vi "robot_ctrl.vi"(2 "Buttons":T1, 3 "Input":T3) -> (1 "Output":T2)   [LabVIEW 2024]
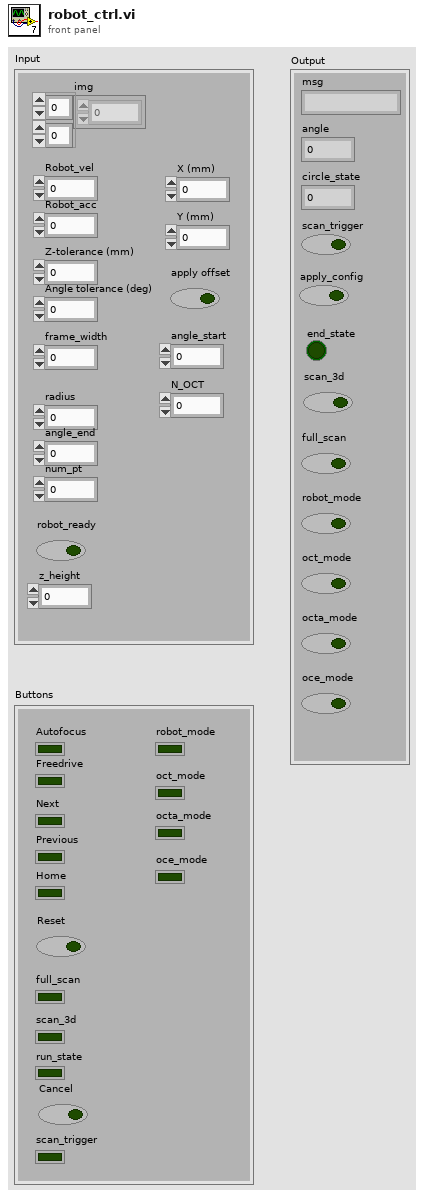
[diagram p1: front panel]
types:
  T1 = cluster{"Autofocus":bool, "Freedrive":bool, "Next":bool, "Previous":bool, "Home":bool, "Reset":bool, "full_scan":bool, "scan_3d":bool, "run_state":bool, "Cancel":bool, "scan_trigger":bool, "robot_mode":bool, "oct_mode":bool, "octa_mode":bool, "oce_mode":bool}
  T2 = cluster{"msg":string, "angle":dbl, "circle_state":i32, "scan_trigger":bool, "apply_config":bool, "end_state":bool, "scan_3d":bool, "full_scan":bool, "robot_mode":bool, "oct_mode":bool, "octa_mode":bool, "oce_mode":bool}
  T3 = cluster{"img":u8[][], "Robot_vel":dbl, "Robot_acc":dbl, "Z-tolerance (mm)":dbl, "Angle tolerance (deg)":dbl, "frame_width":i16, "radius":dbl, "angle_end":dbl, "num_pt":i32, "robot_ready":bool, "z_height":dbl, "X (mm)":dbl, "Y (mm)":dbl, "apply offset":bool, "angle_start":dbl, "N_OCT":i32}
  T4 = cluster{"Robot_vel":dbl, "Robot_acc":dbl, "Z-tolerance (mm)":dbl, "Angle tolerance (deg)":dbl, "radius":dbl, "angle_end":dbl, "num_pt":i32, "z_height":dbl, "Autofocus":bool, "Freedrive":bool, "Next":bool, "Previous":bool, "Home":bool, "Reset":bool, "scan_trigger":bool, "scan_3d":bool, "full_scan":bool, "robot_mode":bool, "oct_mode":bool, "octa_mode":bool, "oce_mode":bool, "X (mm)":dbl, "Y (mm)":dbl, "apply offset":bool, "angle_start":dbl, "N_OCT":i32}
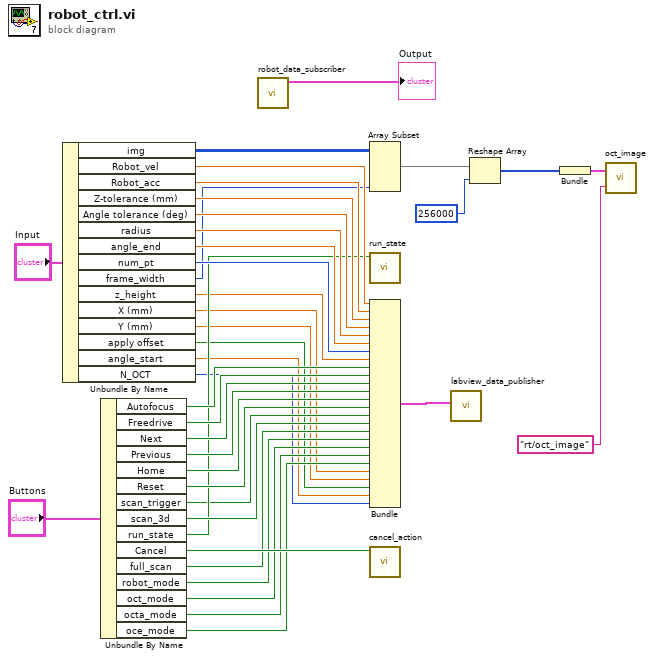
[diagram p0: block diagram]
diagram:
  n1 = Unbundle By Name("Input") -> ("img"=w24:u8[][], "Robot_vel"=w37:dbl, "Robot_acc"=w36:dbl, "Z-tolerance (mm)"=w35:dbl, "Angle tolerance (deg)"=w34:dbl, "radius"=w26:dbl, "angle_end"=w29:dbl, "num_pt"=w28:i32, "frame_width"=w6:i16, "z_height"=w8:dbl, "X (mm)"=w5:dbl, "Y (mm)"=w4:dbl, "apply offset"=w3:bool, "angle_start"=w2:dbl, "N_OCT"=w1:i32)
  n2 = Unbundle By Name("Buttons") -> ("Autofocus"=w25:bool, "Freedrive"=w33:bool, "Next"=w32:bool, "Previous"=w31:bool, "Home"=w30:bool, "Reset"=w27:bool, "scan_trigger"=w14:bool, "scan_3d"=w18:bool, "run_state"=w17:bool, "Cancel"=w15:bool, "full_scan"=w13:bool, "robot_mode"=w12:bool, "oct_mode"=w11:bool, "octa_mode"=w10:bool, "oce_mode"=w9:bool)
  n3 = call "robot_data_subscriber.vi"() -> ("Read Sample"=→"Output":T2)  [unwired: 8 in]
  n4 = Array Subset "Array Subset"(array=w24, length (col)=w6) -> (w22:u8[][])  [unwired: 3 in]
  n5 = call "run_state.vi"("data"=w17) -> ()  [unwired: 11 in]
  n6 = Bundle("Robot_vel"=w37, "Robot_acc"=w36, "Z-tolerance (mm)"=w35, "Angle tolerance (deg)"=w34, "radius"=w26, "angle_end"=w29, "num_pt"=w28, "z_height"=w8, "Autofocus"=w25, "Freedrive"=w33, "Next"=w32, "Previous"=w31, "Home"=w30, "Reset"=w27, "scan_trigger"=w14, "scan_3d"=w18, "full_scan"=w13, "robot_mode"=w12, "oct_mode"=w11, "octa_mode"=w10, "oce_mode"=w9, "X (mm)"=w5, "Y (mm)"=w4, "apply offset"=w3, "angle_start"=w2, "N_OCT"=w1) -> (w7:T4)  [unwired: 1 in]
  n7 = call "cancel_action.vi"("data"=w15) -> ()  [unwired: 11 in]
  n8 = call "labview_data_publisher.vi"("Cluster"=w7) -> ()  [unwired: 10 in]
  n9 = Reshape Array "Reshape Array"(w22, 256000) -> (w19:u8[])
  n10 = Bundle(w19) -> (w20:cluster{u8[]})  [unwired: 1 in]
  n11 = call "oct_image.vi"("topic_name"="rt/oct_image", "img_cluster"=w20) -> ()  [unwired: 1 in]
